vi "12-2-a.vi"(9 "Route in":string[](array[string]), 10 "Start Index":i32, 11 "Array":T1(array[cluster])) -> (1 "Route out":string[][](array[string]))   [LabVIEW 2019, in "12.lvlib"]
uses:
  12.lvlib
  <userlib>/_OpenG.lib/array/array.llb/Remove Duplicates from 1D Array (String)__ogtk.vi
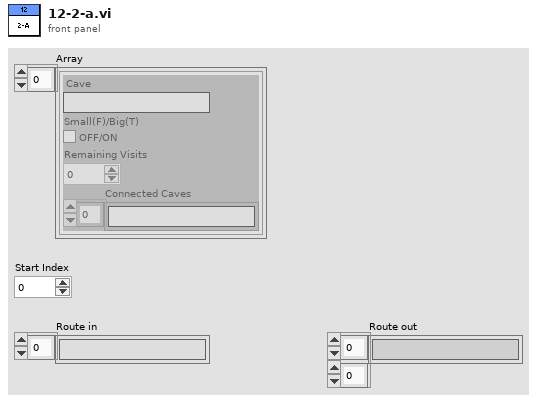
[diagram p1: front panel]
types:
  T1 = cluster{"Cave":string, "Small(F)/Big(T)":bool, "Remaining Visits":i32, "Connected Caves":string[]}[]
  T2 = cluster{"Cave":string, "Small(F)/Big(T)":bool, "Remaining Visits":i32, "Connected Caves":string[]}
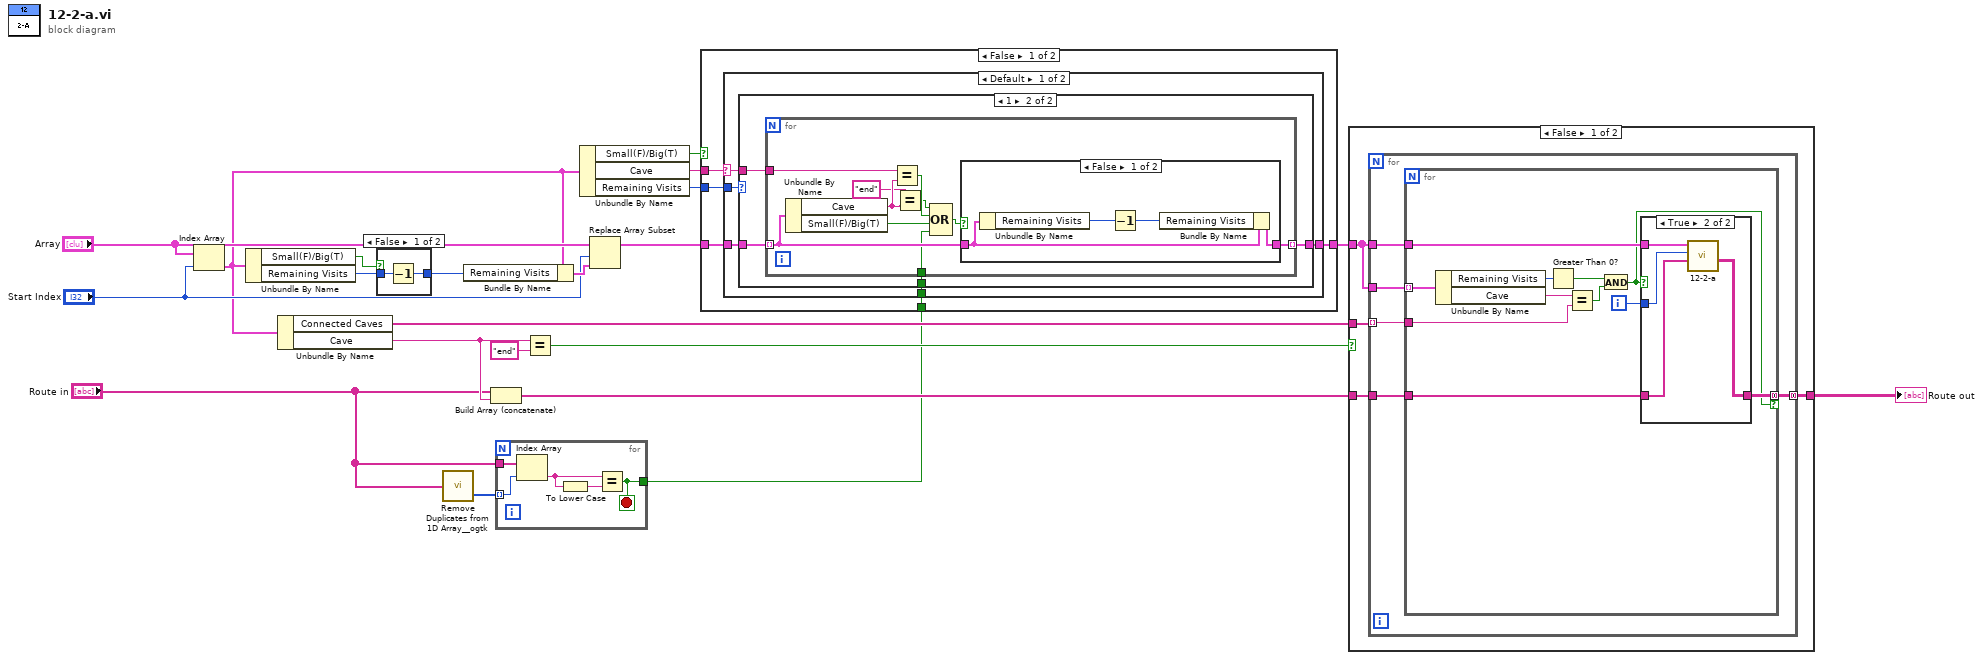
[diagram p0: block diagram]
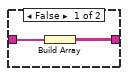
[diagram p7: hidden frame]
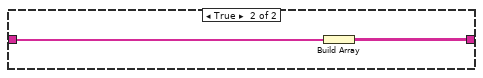
[diagram p8: hidden frame]
diagram:
  n1 = Index Array(array="Array", index="Start Index") -> (element=w7:T2)
  n2 = Unbundle By Name(w7) -> ("Small(F)/Big(T)"=w1:bool, "Remaining Visits"=w6:i32)
  n3 = Unbundle By Name(w7) -> ("Connected Caves"=w21:string[], "Cave"=w15:string)
  n4 = case shown="False" w1 {
    tunnel: w6 -> [w23 w24]
    tunnel: [w22 w24] -> w5
    frame False {
      n5 = Decrement(x=w23) -> (x-1=w22:i32)
    }
    frame True {
    }
  }
  n6 = call-poly <userlib>:"Remove Duplicates from 1D Array__ogtk.vi"("Input Array"="Route in") -> ("indices of removed elements"=w4:i32[])  [unwired: 1 out]
  n7 = Bundle By Name(cluster=w7, "Remaining Visits"=w5) -> (w11:T2)
  n8 = Build Array (concatenate)("Route in", w15) -> (w17:string[])
  n9 = for {
    tunnel: w4 -> [w28] mode=indexing
    tunnel: "Route in" -> [w29]
    tunnel: [w25] -> w3
    stop <- w25 stop-if-true
    n10 = Index Array(array=w29, index=w28) -> (element=w26:string)
    n11 = To Lower Case(string=w26) -> (all lower case string=w27:string)
    n12 = Equal?(x=w26, y=w27) -> (x = y?=w25:bool)
  }
  n13 = Equal?(x=w15, y="end") -> (x = y?=w20:bool)
  n14 = Unbundle By Name(w7) -> ("Small(F)/Big(T)"=w16:bool, "Cave"=w14:string, "Remaining Visits"=w12:i32)
  n15 = Replace Array Subset(array="Array", new element=w11, index="Start Index") -> (w8:T1)
  n16 = case shown="False" w16 {
    tunnel: w14 -> [w31 _]
    tunnel: w12 -> [w34 _]
    tunnel: w8 -> [w33 w61]
    tunnel: [w32 w61] -> w13
    tunnel: w3 -> [w30 _]
    frame False {
      n17 = case shown="Default" w31 {
        selector: w31 -> [w36 _]
        tunnel: w34 -> [w39 _]
        tunnel: w33 -> [w38 w60]
        tunnel: [w37 w60] -> w32
        tunnel: w30 -> [w35 _]
        frame Default {
          n18 = case shown="1" w39 {
            tunnel: w38 -> [w40 w44]
            tunnel: [w40 w43] -> w37
            tunnel: w36 -> [_ w42]
            tunnel: w35 -> [_ w41]
            frame Default {
            }
            frame 1 {
              n19 = for {
                tunnel: w44 -> [w53] mode=indexing
                tunnel: [w52] -> w43 mode=indexing
                tunnel: w42 -> [w50]
                tunnel: w41 -> [w48]
                n20 = Unbundle By Name(w53) -> ("Cave"=w47:string, "Small(F)/Big(T)"=w54:bool)
                n21 = Equal?(x=w50, y=w47) -> (x = y?=w49:bool)
                n22 = Equal?(x="end", y=w47) -> (x = y?=w45:bool)
                n23 = Compound Arithmetic op=OR(w45, w49, w54, w48) -> (w51:bool)
                n24 = case shown="False" w51 {
                  tunnel: w53 -> [w58 w59]
                  tunnel: [w57 w59] -> w52
                  frame False {
                    n25 = Unbundle By Name(w58) -> ("Remaining Visits"=w56:i32)
                    n26 = Decrement(x=w56) -> (x-1=w55:i32)
                    n27 = Bundle By Name(cluster=w58, "Remaining Visits"=w55) -> (w57:T2)
                  }
                  frame True {
                  }
                }
              }
            }
          }
        }
        frame "end", "start" {
        }
      }
    }
    frame True {
    }
  }
  n28 = case shown="False" w20 {
    tunnel: w21 -> [w65 _]
    tunnel: w13 -> [w64 _]
    tunnel: w17 -> [w63 w89]
    tunnel: [w62 w88] -> w18
    frame False {
      n29 = for {
        tunnel: w64 -> [w69]
        tunnel: w65 -> [w70] mode=indexing
        tunnel: w64 -> [w68]
        tunnel: w63 -> [w67]
        tunnel: [w66] -> w62 mode=concatenating
        n30 = for {
          tunnel: w70 -> [w80]
          tunnel: w69 -> [w78] mode=indexing
          tunnel: w68 -> [w77]
          tunnel: w67 -> [w76]
          tunnel: [w74] -> w66 mode=concatenating if=w71
          i -> [w75]
          n31 = Unbundle By Name(w78) -> ("Remaining Visits"=w79:i32, "Cave"=w81:string)
          n32 = Greater Than 0?(x=w79) -> (x > 0?=w72:bool)
          n33 = Equal?(x=w81, y=w80) -> (x = y?=w73:bool)
          n34 = And(x=w72, y=w73) -> (x .and. y?=w71:bool)
          n35 = case shown="True" w71 {
            tunnel: w77 -> [_ w87]
            tunnel: w75 -> [_ w86]
            tunnel: w76 -> [w83 w85]
            tunnel: [w82 w84] -> w74
            frame False {
              n36 = Build Array(w83) -> (w82:string[][])
            }
            frame True {
              n37 = call "12-2-a.vi"("Route in"=w85, "Start Index"=w86, "Array"=w87) -> ("Route out"=w84:string[][])  [unwired: 8 in]
            }
          }
        }
      }
    }
    frame True {
      n38 = Build Array(w89) -> (w88:string[][])
    }
  }
  "Route out" <- w18
